vi "Графики-04-окружность.vi"() -> ()   [LabVIEW 2017]
panel:
  out "XY Graph":cluster{dbl, dbl}[](graph)
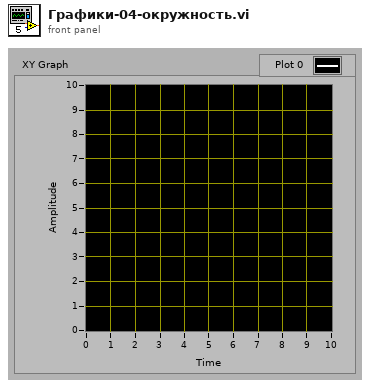
[diagram p1: front panel]
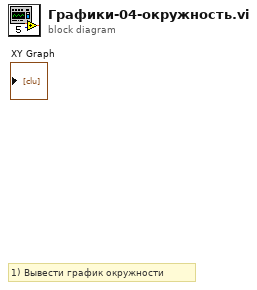
[diagram p0: block diagram]
diagram:
  # "1) Вывести график окружности"
